vi "雷达流速仪全局变量.vi"() -> ()   [LabVIEW 2016, in "雷达流速仪.lvlib"]
uses:
  <vilib>/Plasmionique/MB Master/MB_Master_Serial/MB_Master_Serial.lvclass
panel:
  in  "雷达流速仪类型":string(combo)
  in  "雷达流速仪型号":string
  out "MB_Serial session":refnum<class "MB_Master_Serial.lvclass">
  in  "波特率":u32(ring)=9600 items=["9600"=9600, "19200"=19200, "115200"=115200]
  in  "雷达流速仪串口":refnum<visa-resource-name>="COM6"
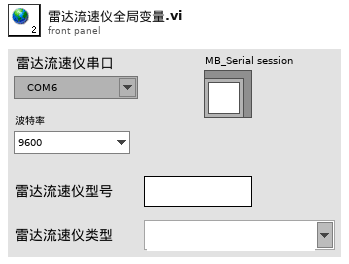
[diagram p1: front panel]
diagram:
